vi "Simple Add.vi"() -> ()   [LabVIEW 2018]
panel:
  out "Sum":dbl
  in  "Addend  3":dbl
  in  "Addend 1":dbl
  in  "Added 2":dbl
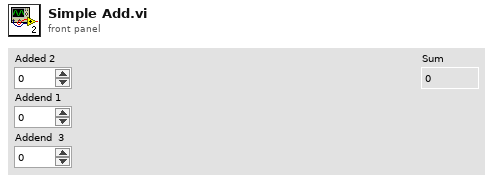
[diagram p1: front panel]
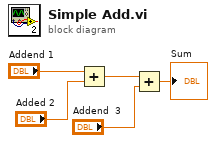
[diagram p0: block diagram]
diagram:
  n1 = Add(x="Addend 1", y="Added 2") -> (x+y=w3:dbl)
  n2 = Add(x=w3, y="Addend  3") -> (x+y=→"Sum":dbl)
